vi "formatPath.vi"(9 "Value":path, 11 "StringFormatter":refnum<class "StringFormatter.lvclass">) -> (1 "Formatted Value":string)   [LabVIEW 2020, in "OpenStringFormatter.lvlib" / "StringFormatter.lvclass"]
uses:
  StringFormatter.lvclass
  StringFormatter.lvclass/StringFormatter.ctl
  _built_ppls/OpenConvert.lvlibp
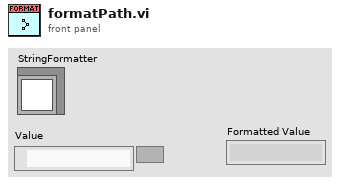
[diagram p1: front panel]
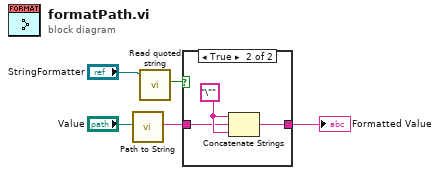
[diagram p0: block diagram]
diagram:
  n1 = call "Path to String.vi"("specific path"="Value") -> ("common path"=w1:string)  [unwired: 10 in]
  n2 = call "Read quoted string.vi"("StringFormatter in"="StringFormatter") -> ("quoted string"=w5:bool)  [unwired: 9 in, 1 out]
  n3 = case shown="True" w5 {
    tunnel: [w6 w8] -> w3
    tunnel: w1 -> [w6 w7]
    frame False {
    }
    frame True {
      w9 = "\"" ("string")
      n4 = Concatenate Strings(w9, w7, w9) -> (w8:string)
    }
  }
  "Formatted Value" <- w3
